vi "Load Products.vi"(8 "error in (no error)":errorcluster, 11 "Products Picker in":refnum<class "Products Picker.lvclass">) -> (0 "error out":errorcluster, 3 "Products Picker out":refnum<class "Products Picker.lvclass">)   [LabVIEW 2020, in "Products Picker.lvlib" / "Products Picker.lvclass"]
uses:
  Products Picker.lvclass
  Products Picker.lvclass/Products Picker.ctl
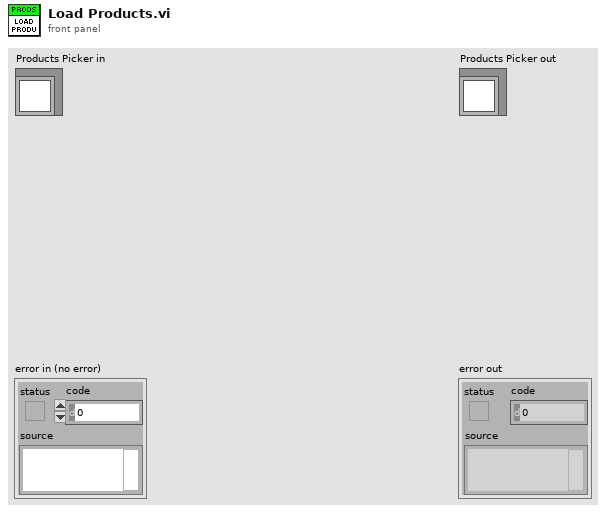
[diagram p1: front panel]
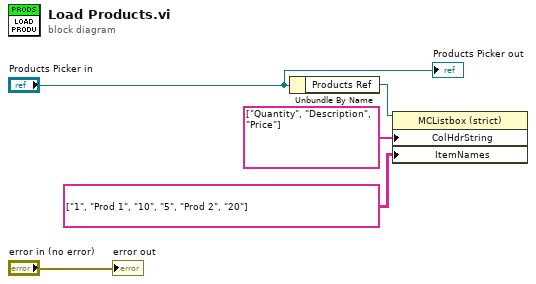
[diagram p0: block diagram]
diagram:
  n1 = Unbundle By Name("Products Picker in") -> ("Products Ref"=w3:refnum<vi>)
  n2 = property class="MCListbox (strict)"(reference=w3, "ColHdrString"=string[] ["Quantity", "Description", "Price"] ("Column Header Strings[]"), "ItemNames"=string[][] [["1", "Prod 1", "10"], ["5", "Prod 2", "20"]] ("Item Names")) -> ()  [unwired: 1 in, 2 out]
  "error out" <- "error in (no error)"
  "Products Picker out" <- "Products Picker in"
